vi "Login_window.vi"(0 "vi path":path) -> (4 "vi path 2":path)   [LabVIEW 2011]
uses:
  <vilib>/Utility/file.llb/Read From Spreadsheet File (string).vi
  <vilib>/Utility/file.llb/Write To Spreadsheet File (string).vi
panel:
  out "resolution_y":i16
  out "resolution":i16
  in  "Input Device":enum32{"Mouse", "Wii Mote", "Kinect"}(radio)
  in  "Last Name":string
  out "vi path 4":path
  in  "vi path 3":path
  out "Skip":bool
  out "Contents":string[][](array[string])
  in  "Cancel":bool
  in  "OK Button":bool
  in  "First Name":string
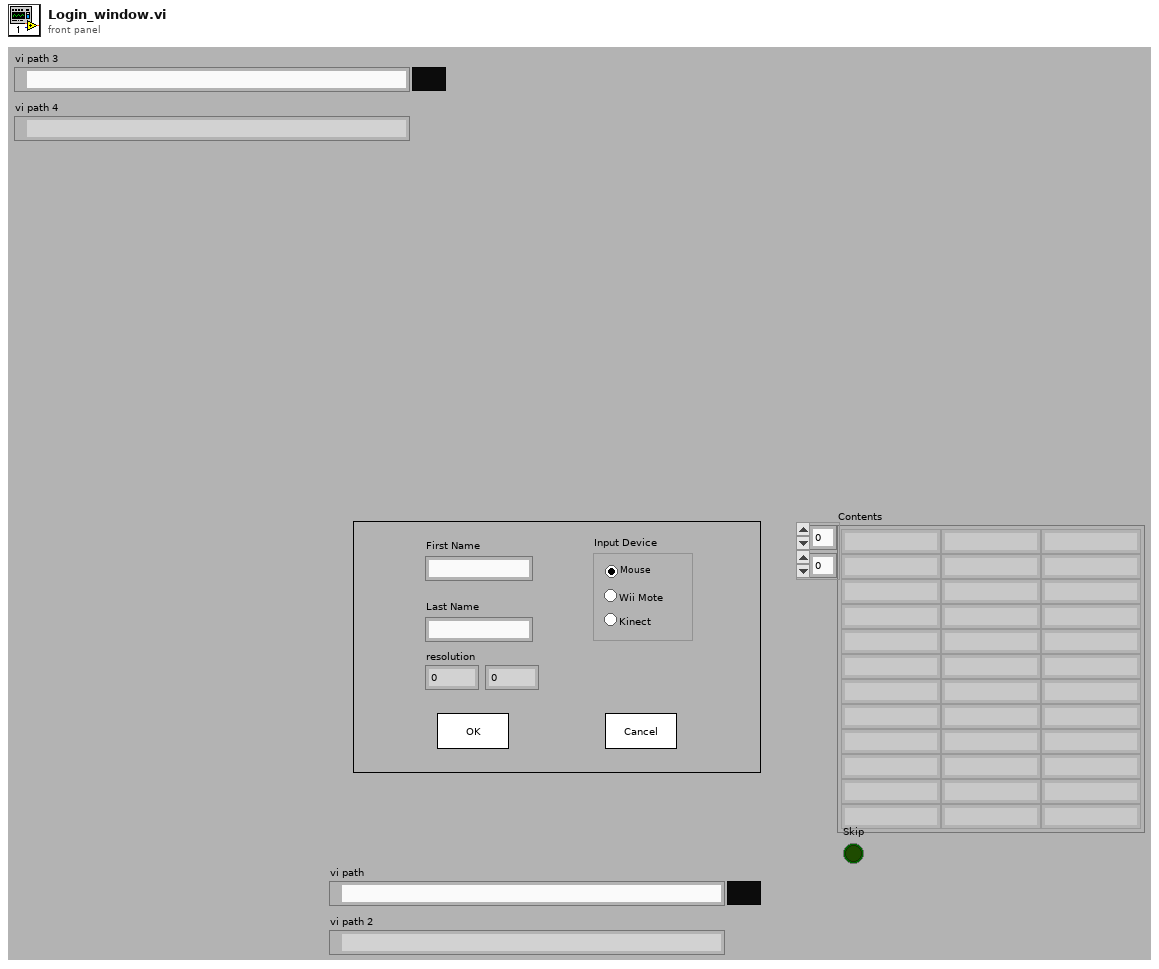
[diagram p1: front panel]
types:
  T1 = enum16{"open", "open or create", "create or replace", "create", "open (read only)"}
  T2 = typedef "LVAllMonitorsDisplayTypeDef.ctl" = cluster{"Bounds":cluster{"Left":i16, "Top":i16, "Right":i16, "Bottom":i16}, "Depth":i16}[]
  T3 = cluster{"Bounds":cluster{"Left":i16, "Top":i16, "Right":i16, "Bottom":i16}, "Depth":i16}
  T4 = cluster{"Left":i16, "Top":i16, "Right":i16, "Bottom":i16}
  T5 = enum16{"open", "replace", "create", "open or create", "replace or create", "replace or create with confirmation"}
  T6 = enum16{"Left Button", "Center Button", "Right Button", "Window Close"}
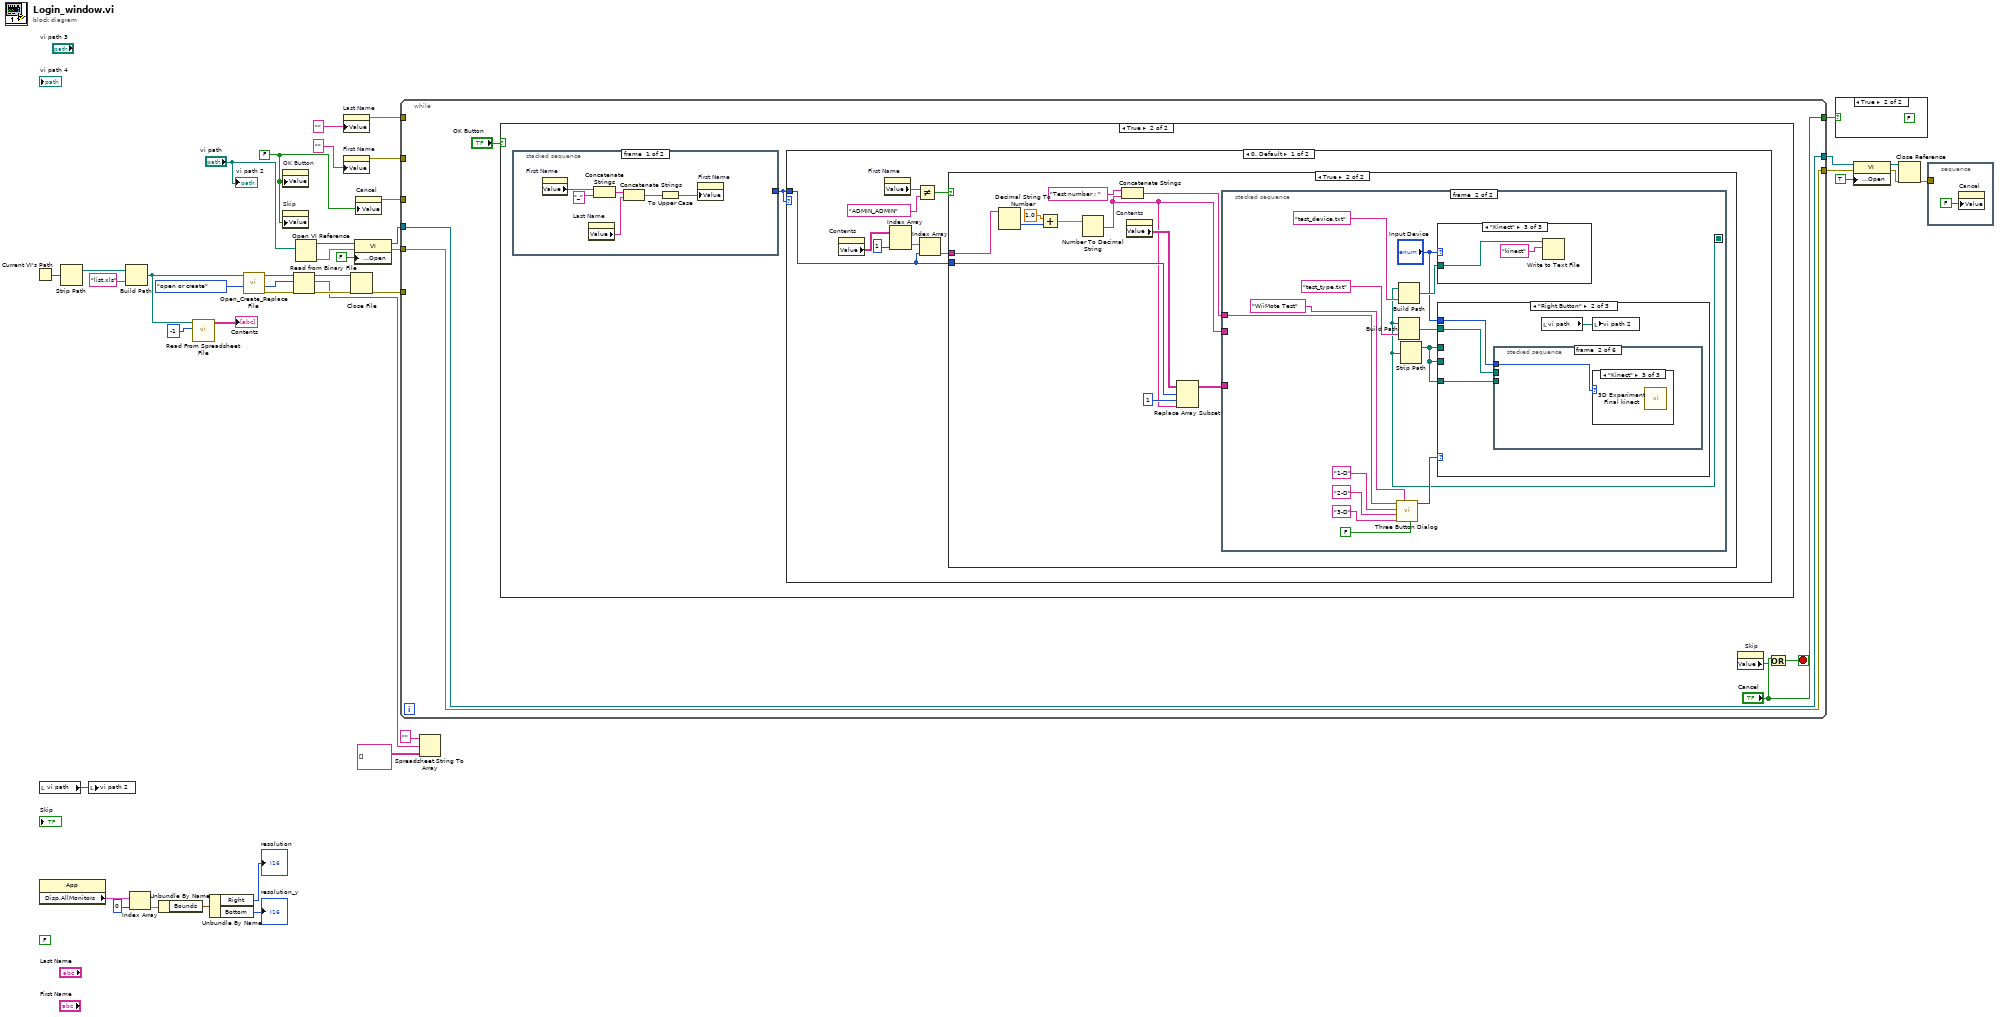
[diagram p0: block diagram]
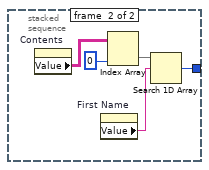
[diagram p4: hidden frame]
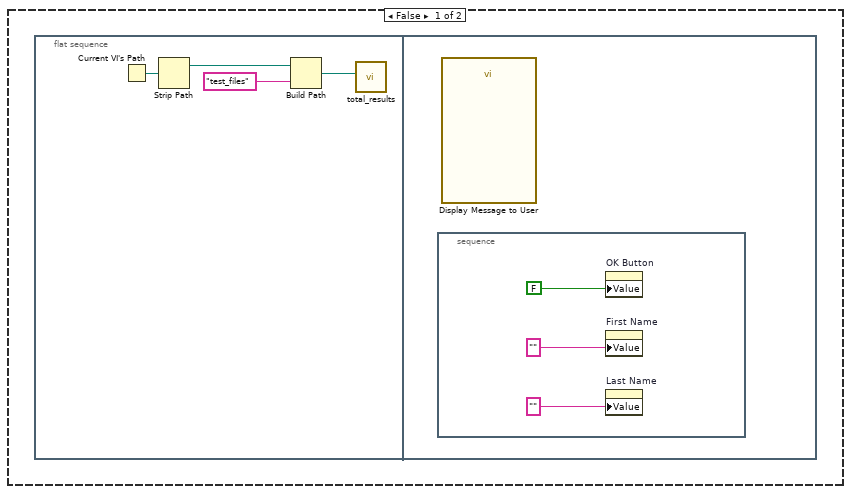
[diagram p5: hidden frame]
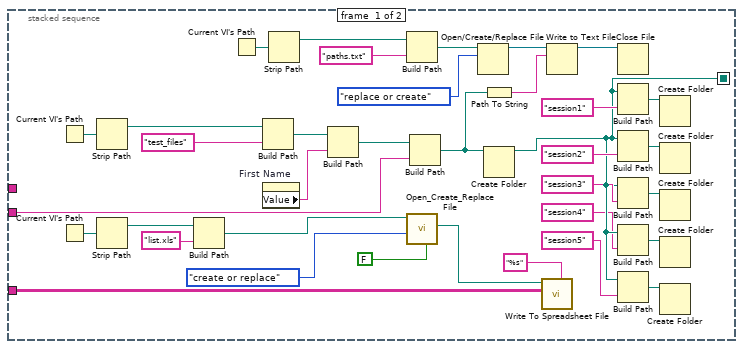
[diagram p6: hidden frame]
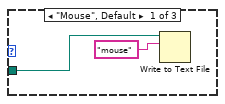
[diagram p7: hidden frame]
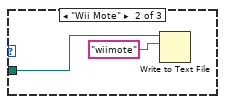
[diagram p8: hidden frame]
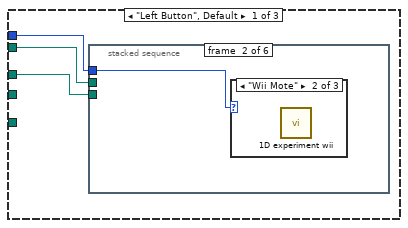
[diagram p9: hidden frame]
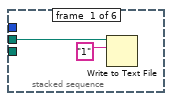
[diagram p10: hidden frame]
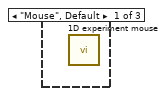
[diagram p11: hidden frame]
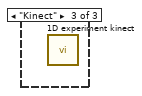
[diagram p12: hidden frame]
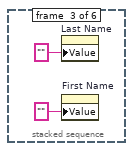
[diagram p13: hidden frame]
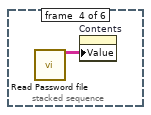
[diagram p14: hidden frame]
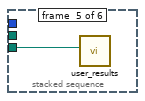
[diagram p15: hidden frame]
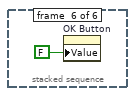
[diagram p16: hidden frame]
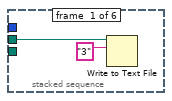
[diagram p17: hidden frame]
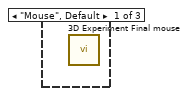
[diagram p18: hidden frame]
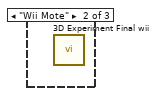
[diagram p19: hidden frame]
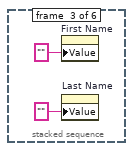
[diagram p20: hidden frame]
diagram:
  w18 = FALSE ("true")
  (unwired) FALSE ("true")
  n1 = Current VI's Path() -> (path=w16:path)
  n2 = local read "vi path"() -> (w22:path)
  n3 = property class="App"() -> ("Disp.AllMonitors"=w4:T2)  [unwired: 2 in, 2 out]
  n4 = Strip Path(path=w16) -> (stripped path=w15:path)  [unwired: 1 out]
  n5 = local write "vi path 2"(w22) -> ()
  n6 = Build Path(base path=w15, name or relative path="list.xls") -> (appended path=w11:path)
  n7 = Index Array(array=w4, index=u16 0 ("Front Panel Window:Monitor")) -> (element=w6:T3)
  n8 = Unbundle By Name(w6) -> ("Bounds"=w3:T4)
  n9 = call-poly <vilib>:"Read From Spreadsheet File.vi"("number of rows (all:-1)"=-1, "file path (dialog if empty)"=w11) -> ("all rows"=→"Contents":string[][])  [unwired: 5 in, 4 out]
  n10 = Unbundle By Name(w3) -> ("Right"=→"resolution":i16, "Bottom"=→"resolution_y":i16)
  n11 = call <vilib>:"Open_Create_Replace File.vi"("function (open:0)"=T1."open or create", "file path"=w11) -> ("error out"=w42:errorcluster, "file size (bytes)"=w38:i32, "refnum"=w41:refnum<file>)  [unwired: 6 in, 1 out]
  n12 = property on="OK Button" class="Bool (strict)"("Value"=w18) -> ()  [unwired: 2 in, 2 out]
  n13 = property on="Skip" class="Bool (strict)"("Value"=w18) -> ()  [unwired: 2 in, 2 out]
  n14 = Read from Binary File(8:w42, 10:w38, 11:w41) -> (0:w40:errorcluster, 2:w37:string, 3:w39:refnum<file>)  [unwired: 3 in, 1 out]
  n15 = Open VI Reference(vi path="vi path") -> (vi reference=w32:refnum<vi>, error out=w31:errorcluster)  [unwired: 5 in]
  n16 = property on="Last Name" class="Str"("Value"="" ("User Name")) -> (error out=w7:errorcluster)  [unwired: 2 in, 1 out]
  n17 = property on="First Name" class="Str"("Value"="" ("User Name")) -> (error out=w12:errorcluster)  [unwired: 2 in, 1 out]
  n18 = Close File(refnum=w39, error in=w40) -> (error out=w35:errorcluster)  [unwired: 1 out]
  n19 = property class="VI"(reference=w32, error in=w31, "Front Panel Window:Open"=FALSE) -> (reference out=w29:refnum<vi>, error out=w28:errorcluster)
  n20 = property on="Cancel" class="Bool (strict)"("Value"=w18) -> (error out=w21:errorcluster)  [unwired: 2 in, 1 out]
  n21 = while {
    tunnel: w35 -> [_]
    tunnel: w29 -> [w47]
    tunnel: w28 -> [w46]
    tunnel: [w47] -> w26
    tunnel: [w46] -> w25
    tunnel: w21 -> [_]
    tunnel: ["Cancel"] -> w19
    tunnel: w12 -> [_]
    tunnel: w7 -> [_]
    stop <- w43 stop-if-true
    n22 = case shown="True" "OK Button" {
      frame False {
      }
      frame True {
        n23 = stacked-sequence {
          tunnel: [_ w56] -> w49
          frame #0 {
            n24 = property on="First Name" class="Str"() -> ("Value"=w54:string)  [unwired: 2 in, 2 out]
            n25 = property on="Last Name" class="Str"() -> ("Value"=w53:string)  [unwired: 2 in, 2 out]
            n26 = Concatenate Strings(w54, "_" ("string")) -> (w52:string)
            n27 = Concatenate Strings(w52, w53) -> (w51:string)
            n28 = To Upper Case(1:w51) -> (0:w50:string)
            n29 = property on="First Name" class="Str"("Value"=w50) -> ()  [unwired: 2 in, 2 out]
          }
          frame #1 {
            n30 = property on="Contents" class="Arr (strict)"() -> ("Value"=w58:string[][])  [unwired: 2 in, 2 out]
            n31 = property on="First Name" class="Str"() -> ("Value"=w57:string)  [unwired: 2 in, 2 out]
            n32 = Index Array(array=w58, index (col)=0 ("disabled index (col)")) -> (element=w60:string[])  [unwired: 1 in]
            n33 = Search 1D Array(1D array=w60, element=w57) -> (index of element=w56:i32)  [unwired: 1 in]
          }
        }
        n34 = case shown="0, Default" w49 {
          tunnel: w49 -> [w63 _]
          frame 0, Default {
            n35 = property on="Contents" class="Arr (strict)"() -> ("Value"=w67:string[][])  [unwired: 2 in, 2 out]
            n36 = property on="First Name" class="Str"() -> ("Value"=w65:string)  [unwired: 2 in, 2 out]
            n37 = Index Array(array=w67, index (col)=1 ("disabled index (col)")) -> (element=w66:string[])  [unwired: 1 in]
            n38 = Not Equal?(x=w65, y="ADMIN_ADMIN") -> (x != y?=w61:bool)
            n39 = Index Array(array=w66, index=w63) -> (element=w62:string)
            n40 = case shown="True" w61 {
              tunnel: w63 -> [_ w82]
              tunnel: w62 -> [_ w78]
              frame False {
                n41 = flat-sequence {
                  frame #0 {
                    n42 = Current VI's Path() -> (path=w72:path)
                    n43 = Strip Path(path=w72) -> (stripped path=w70:path)  [unwired: 1 out]
                    n44 = Build Path(base path=w70, name or relative path="test_files") -> (appended path=w71:path)
                    n45 = call "total_results.vi"("Users Path"=w71) -> ()  [unwired: 11 in]
                  }
                  frame #1 {
                    n46 = stacked-sequence {
                      frame #0 {
                        n47 = property on="OK Button" class="Bool (strict)"("Value"=FALSE ("true")) -> ()  [unwired: 2 in, 2 out]
                        n48 = property on="First Name" class="Str"("Value"="" ("User Name")) -> ()  [unwired: 2 in, 2 out]
                        n49 = property on="Last Name" class="Str"("Value"="" ("User Name")) -> ()  [unwired: 2 in, 2 out]
                      }
                    }
                    n50 = call "Display Message to User"() -> ()  [unwired: 10 in, 2 out]
                  }
                }
              }
              frame True {
                n51 = Decimal String To Number(string=w78) -> (number=w84:i32)  [unwired: 2 in, 1 out]
                n52 = Add(x=1.0, y=w84) -> (x+y=w83:dbl)
                n53 = Number To Decimal String(number=w83) -> (decimal integer string=w76:string)  [unwired: 1 in]
                n54 = Concatenate Strings("Test number : " ("message"), w76) -> (w77:string)
                n55 = property on="Contents" class="Arr (strict)"() -> ("Value"=w86:string[][])  [unwired: 2 in, 2 out]
                n56 = Replace Array Subset(array=w86, new element=w76, index (row)=w82, index (col)=1 ("disabled index (col)")) -> (w80:string[][])
                n57 = stacked-sequence {
                  seq-local: [w89 _] -> [_ w125]
                  tunnel: w80 -> [w115 _]
                  tunnel: w77 -> [_ w131]
                  tunnel: w76 -> [w103 _]
                  frame #0 {
                    n58 = Current VI's Path() -> (path=w110:path)
                    n59 = Current VI's Path() -> (path=w120:path)
                    n60 = Strip Path(path=w110) -> (stripped path=w108:path)  [unwired: 1 out]
                    n61 = Strip Path(path=w120) -> (stripped path=w119:path)  [unwired: 1 out]
                    n62 = Build Path(base path=w119, name or relative path="list.xls") -> (appended path=w117:path)
                    n63 = Current VI's Path() -> (path=w102:path)
                    n64 = Build Path(base path=w108, name or relative path="test_files") -> (appended path=w107:path)
                    n65 = property on="First Name" class="Str"() -> ("Value"=w109:string)  [unwired: 2 in, 2 out]
                    n66 = Strip Path(path=w102) -> (stripped path=w101:path)  [unwired: 1 out]
                    n67 = Build Path(base path=w107, name or relative path=w109) -> (appended path=w105:path)
                    n68 = Build Path(base path=w101, name or relative path="paths.txt") -> (appended path=w99:path)
                    n69 = call <vilib>:"Open_Create_Replace File.vi"("advisory dialog? (display:T)"=FALSE, "function (open:0)"=T1."create or replace", "file path"=w117) -> ("new file path"=w116:path)  [unwired: 5 in, 3 out]
                    n70 = Build Path(base path=w105, name or relative path=w103) -> (appended path=w104:path)
                    n71 = Open/Create/Replace File(file path (use dialog)=w99, operation (0:open)=T5."replace or create") -> (refnum out=w111:refnum<file>)  [unwired: 4 in, 2 out]
                    n72 = Path To String(path=w104) -> (string=w92:string)
                    n73 = Create Folder(path (use dialog)=w104) -> (created path=w89:path)  [unwired: 2 in, 2 out]
                    n74 = call-poly <vilib>:"Write To Spreadsheet File.vi"("format (%s)"="%s", "2D data"=w115, "file path (dialog if empty)"=w116) -> ()  [unwired: 5 in, 1 out]
                    n75 = Write to Text File(file (use dialog)=w111, text=w92) -> (refnum out=w112:refnum<file>)  [unwired: 2 in, 2 out]
                    n76 = Close File(refnum=w112) -> ()  [unwired: 1 in, 2 out]
                    n77 = Build Path(base path=w89, name or relative path="session1") -> (appended path=w97:path)
                    n78 = Build Path(base path=w89, name or relative path="session2") -> (appended path=w95:path)
                    n79 = Build Path(base path=w89, name or relative path="session3") -> (appended path=w96:path)
                    n80 = Build Path(base path=w89, name or relative path="session4") -> (appended path=w91:path)
                    n81 = Build Path(base path=w89, name or relative path="session5") -> (appended path=w90:path)
                    n82 = Create Folder(path (use dialog)=w97) -> ()  [unwired: 2 in, 3 out]
                    n83 = Create Folder(path (use dialog)=w95) -> ()  [unwired: 2 in, 3 out]
                    n84 = Create Folder(path (use dialog)=w96) -> ()  [unwired: 2 in, 3 out]
                    n85 = Create Folder(path (use dialog)=w91) -> ()  [unwired: 2 in, 3 out]
                    n86 = Create Folder(path (use dialog)=w90) -> ()  [unwired: 2 in, 3 out]
                  }
                  frame #1 {
                    n87 = call <vilib>:"Three Button Dialog.vi"("Allow user to close window? (TRUE)"=FALSE, "Window Title (\"\")"="WiiMote Test" ("Window Title (\"\")"), "Right Button Text (\"Cancel\")"="3-D" ("Left Button Text (\"Yes\")"), "Center Button Text (\"No\")"="2-D" ("Left Button Text (\"Yes\")"), "Left Button Text (\"Yes\")"="1-D" ("Left Button Text (\"Yes\")"), "message"=w131) -> ("Which Button?"=w132:T6)  [unwired: 5 in]
                    n88 = Build Path(base path=w125, name or relative path="test_device.txt") -> (appended path=w126:path)
                    n89 = Build Path(base path=w125, name or relative path="test_type.txt") -> (appended path=w128:path)
                    n90 = Strip Path(path=w125) -> (stripped path=w124:path)  [unwired: 1 out]
                    n91 = case shown="\"Kinect\"" "Input Device" {
                      tunnel: w126 -> [w137 w139 w141]
                      frame "Mouse", Default {
                        n92 = Write to Text File(file (use dialog)=w137, text="mouse") -> ()  [unwired: 2 in, 3 out]
                      }
                      frame "Wii Mote" {
                        n93 = Write to Text File(file (use dialog)=w139, text="wiimote") -> ()  [unwired: 2 in, 3 out]
                      }
                      frame "Kinect" {
                        n94 = Write to Text File(file (use dialog)=w141, text="kinect") -> ()  [unwired: 2 in, 3 out]
                      }
                    }
                    n95 = case shown="\"Right Button\"" w132 {
                      tunnel: w128 -> [w145 w156 w168]
                      tunnel: w124 -> [_ _ w167]
                      tunnel: w124 -> [w144 _ _]
                      tunnel: w124 -> [_ w155 _]
                      tunnel: "Input Device" -> [w143 w154 w166]
                      frame "Left Button", Default {
                        n96 = stacked-sequence {
                          tunnel: w145 -> [w146 _ _ _ _ _]
                          tunnel: w144 -> [_ _ _ _ w152 _]
                          tunnel: w143 -> [_ w148 _ _ _ _]
                          frame #0 {
                            n97 = Write to Text File(file (use dialog)=w146, text="1") -> ()  [unwired: 2 in, 3 out]
                          }
                          frame #1 {
                            n98 = case shown="\"Wii Mote\"" w148 {
                              frame "Mouse", Default {
                                n99 = call "1D experiment mouse.vi"() -> ()  [unwired: 12 in]
                              }
                              frame "Wii Mote" {
                                n100 = call "1D experiment wii.vi"() -> ()  [unwired: 12 in]
                              }
                              frame "Kinect" {
                                n101 = call "1D experiment kinect.vi"() -> ()  [unwired: 12 in]
                              }
                            }
                          }
                          frame #2 {
                            n102 = property on="Last Name" class="Str"("Value"="" ("Password")) -> ()  [unwired: 2 in, 2 out]
                            n103 = property on="First Name" class="Str"("Value"="" ("Password")) -> ()  [unwired: 2 in, 2 out]
                          }
                          frame #3 {
                            n104 = call "Read Password file.vi"() -> ("Contents"=w151:string[][])  [unwired: 15 in]
                            n105 = property on="Contents" class="Arr (strict)"("Value"=w151) -> ()  [unwired: 2 in, 2 out]
                          }
                          frame #4 {
                            n106 = call "user_results.vi"("user path"=w152) -> ()  [unwired: 11 in]
                          }
                          frame #5 {
                            n107 = property on="OK Button" class="Bool (strict)"("Value"=FALSE ("true")) -> ()  [unwired: 2 in, 2 out]
                          }
                        }
                      }
                      frame "Right Button" {
                        n108 = stacked-sequence {
                          tunnel: w156 -> [w158 _ _ _ _ _]
                          tunnel: w155 -> [_ _ _ _ w164 _]
                          tunnel: w154 -> [_ w160 _ _ _ _]
                          frame #0 {
                            n109 = Write to Text File(file (use dialog)=w158, text="3") -> ()  [unwired: 2 in, 3 out]
                          }
                          frame #1 {
                            n110 = case shown="\"Kinect\"" w160 {
                              frame "Mouse", Default {
                                n111 = call "3D Experiment Final mouse.vi"() -> ()  [unwired: 12 in]
                              }
                              frame "Wii Mote" {
                                n112 = call "3D Experiment Final wii.vi"() -> ()  [unwired: 12 in]
                              }
                              frame "Kinect" {
                                n113 = call "3D Experiment Final kinect.vi"() -> ()  [unwired: 12 in]
                              }
                            }
                          }
                          frame #2 {
                            n114 = property on="First Name" class="Str"("Value"="" ("Password")) -> ()  [unwired: 2 in, 2 out]
                            n115 = property on="Last Name" class="Str"("Value"="" ("Password")) -> ()  [unwired: 2 in, 2 out]
                          }
                          frame #3 {
                            n116 = call "Read Password file.vi"() -> ("Contents"=w163:string[][])  [unwired: 15 in]
                            n117 = property on="Contents" class="Arr (strict)"("Value"=w163) -> ()  [unwired: 2 in, 2 out]
                          }
                          frame #4 {
                            n118 = call "user_results.vi"("user path"=w164) -> ()  [unwired: 11 in]
                          }
                          frame #5 {
                            n119 = property on="OK Button" class="Bool (strict)"("Value"=FALSE ("true")) -> ()  [unwired: 2 in, 2 out]
                          }
                        }
                        n120 = local read "vi path"() -> (w157:path)
                        n121 = local write "vi path 2"(w157) -> ()
                      }
                      frame "Center Button" {
                        n122 = stacked-sequence {
                          tunnel: w168 -> [w170 _ _ _ _ _]
                          tunnel: w167 -> [_ _ _ _ w175 _]
                          tunnel: w166 -> [_ w171 _ _ _ _]
                          frame #0 {
                            n123 = Write to Text File(file (use dialog)=w170, text="2") -> ()  [unwired: 2 in, 3 out]
                          }
                          frame #1 {
                            n124 = case shown="\"Wii Mote\"" w171 {
                              frame "Mouse", Default {
                                n125 = call "2D experiment mouse.vi"() -> ()  [unwired: 12 in]
                              }
                              frame "Wii Mote" {
                                n126 = call "2D experiment wii.vi"() -> ()  [unwired: 12 in]
                              }
                              frame "Kinect" {
                                n127 = call "2D experiment kinect.vi"() -> ()  [unwired: 12 in]
                              }
                            }
                          }
                          frame #2 {
                            n128 = property on="First Name" class="Str"("Value"="" ("Password")) -> ()  [unwired: 2 in, 2 out]
                            n129 = property on="Last Name" class="Str"("Value"="" ("Password")) -> ()  [unwired: 2 in, 2 out]
                          }
                          frame #3 {
                            n130 = call "Read Password file.vi"() -> ("Contents"=w174:string[][])  [unwired: 15 in]
                            n131 = property on="Contents" class="Arr (strict)"("Value"=w174) -> ()  [unwired: 2 in, 2 out]
                          }
                          frame #4 {
                            n132 = call "user_results.vi"("user path"=w175) -> ()  [unwired: 11 in]
                          }
                          frame #5 {
                            n133 = property on="OK Button" class="Bool (strict)"("Value"=FALSE ("true")) -> ()  [unwired: 2 in, 2 out]
                          }
                        }
                      }
                    }
                  }
                }
              }
            }
          }
          frame -1 {
            n134 = stacked-sequence {
              seq-local: [w177 _ _ _] -> [_ w181 _ _]
              frame #0 {
                n135 = property on="First Name" class="Str"() -> ("Value"=w180:string)  [unwired: 2 in, 2 out]
                n136 = Build Array(w180, "0" ("element"), "user") -> (w177:string[])
              }
              frame #1 {
                n137 = property on="Contents" class="Arr (strict)"() -> ("Value"=w183:string[][])  [unwired: 2 in, 2 out]
                n138 = Insert Into Array(array=w183, new element=w181) -> (w182:string[][])  [unwired: 2 in]
                n139 = property on="Contents" class="Arr (strict)"("Value"=w182) -> ()  [unwired: 2 in, 2 out]
              }
              frame #2 {
                n140 = Current VI's Path() -> (path=w188:path)
                n141 = Strip Path(path=w188) -> (stripped path=w187:path)  [unwired: 1 out]
                n142 = Build Path(base path=w187, name or relative path="list.xls") -> (appended path=w185:path)
                n143 = property on="Contents" class="Arr (strict)"() -> ("Value"=w194:string[][])  [unwired: 2 in, 2 out]
                n144 = Array To Spreadsheet String(array=w194, 3:"%s" ("format string")) -> (spreadsheet string=w193:string)  [unwired: 1 in]
                n145 = call <vilib>:"Open_Create_Replace File.vi"("advisory dialog? (display:T)"=FALSE, "function (open:0)"=T1."create or replace", "file path"=w185) -> ("error out"=w195:errorcluster, "refnum"=w196:refnum<file>)  [unwired: 5 in, 2 out]
                n146 = Write to Binary File(file (use dialog)=w196, data=w193, error in=w195, 5:FALSE ("prepend array or string size? (T)")) -> (refnum out=w189:refnum<file>, error out=w190:errorcluster)  [unwired: 2 in, 1 out]
                n147 = Close File(refnum=w189, error in=w190) -> ()  [unwired: 2 out]
              }
              frame #3 {
                n148 = One Button Dialog(message="User Created") -> (true=w198:bool)  [unwired: 1 in]
                n149 = stacked-sequence {
                  tunnel: w198 -> [_]
                  frame #0 {
                    n150 = property on="OK Button" class="Bool (strict)"("Value"=FALSE ("true")) -> ()  [unwired: 2 in, 2 out]
                    n151 = property on="First Name" class="Str"("Value"="" ("Password")) -> ()  [unwired: 2 in, 2 out]
                    n152 = property on="Last Name" class="Str"("Value"="" ("Password")) -> ()  [unwired: 2 in, 2 out]
                  }
                }
              }
            }
          }
        }
      }
    }
    n153 = property on="Skip" class="Bool (strict)"() -> ("Value"=w44:bool)  [unwired: 2 in, 2 out]
    n154 = Or(x="Cancel", y=w44) -> (x .or. y?=w43:bool)
  }
  n155 = Spreadsheet String To Array(format string="", spreadsheet string=w37, array type (2D Dbl)=string[][] []) -> ()  [unwired: 1 in, 1 out]
  n156 = case shown="True" w19 {
    frame False {
    }
    frame True {
      (unwired) FALSE ("true")
    }
  }
  n157 = property class="VI"(reference=w26, error in=w25, "Front Panel Window:Open"=TRUE) -> (reference out=w24:refnum<vi>, error out=w23:errorcluster)
  n158 = Close Reference(reference=w24, error in (no error)=w23) -> (error out=w20:errorcluster)
  n159 = stacked-sequence {
    tunnel: w20 -> [_]
    frame #0 {
      n160 = property on="Cancel" class="Bool (strict)"("Value"=FALSE ("true")) -> ()  [unwired: 2 in, 2 out]
    }
  }
  "vi path 2" <- "vi path"
